vi "Check_Running.vi"(0 "connection ID":refnum<k5>, 3 "error in (no error)":errorcluster) -> (5 "Velocity":dbl, 7 "connection ID out":refnum<k5>, 8 "Status":bool, 9 "Motor Status":string, 10 "error out":errorcluster)   [LabVIEW 2019]
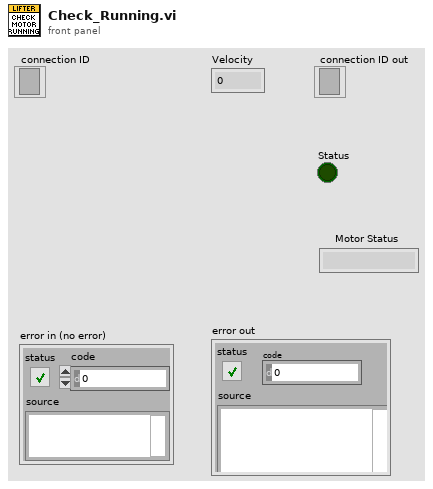
[diagram p1: front panel]
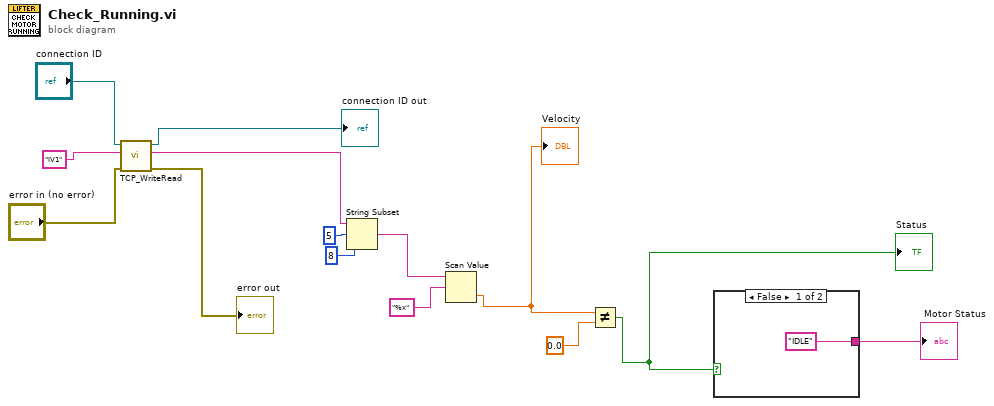
[diagram p0: block diagram]
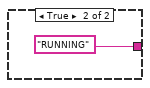
[diagram p2: hidden frame]
diagram:
  n1 = call "TCP_WriteRead.vi"("error in"="error in (no error)", "Parameter 1"="IV1" ("string"), "connection ID"="connection ID") -> ("error out"=→"error out":errorcluster, "DataOut"=w2:string, "TCP Network Connection out"=→"connection ID out":refnum<k5>)  [unwired: 6 in]
  n2 = String Subset(string=w2, offset (0)=5, length (rest)=8 ("length (rest)")) -> (substring=w7:string)
  n3 = Scan Value(string=w7, format string="%x") -> (value=w11:dbl)  [unwired: 1 in, 1 out]
  "Velocity" <- w11
  n4 = Not Equal?(x=w11, y=0.0) -> (x != y?=w9:bool)
  "Status" <- w9
  n5 = case shown="False" w9 {
    tunnel: ["IDLE" ("Motor") "RUNNING" ("Motor")] -> w8
    frame False {
    }
    frame True {
    }
  }
  "Motor Status" <- w8
